vi "openCOMports.vi"(1 "COM Port":refnum<visa-resource-name>="COM8", 2 "index":i32) -> (0 "opened COM port":refnum<visa-resource-name>="COM8")   [LabVIEW 2015]
uses:
  <vilib>/Instr/_visa.llb/VISA Configure Serial Port (Instr).vi
panel:
  in  "Comms":T1(array[cluster])=[{"baud rate "=500000, "data bits "=8, "parity "=enum."None", "flow control "=0, "timeout "=10000, "stop bits "=10}, {"baud rate "=57600, "data bits "=8, "parity "=enum."None", "flow control "=0, "timeout "=10000, "stop bits "=10}] {"stop bits" items=["1.0"=10, "1.5"=15, "2.0"=20]; "flow control" items=["None", "XON/XOFF", "RTS/CTS", "XON/XOFF & RTS/CTS", "DTR/DSR", "XON/XOFF & DTR/DSR"]}
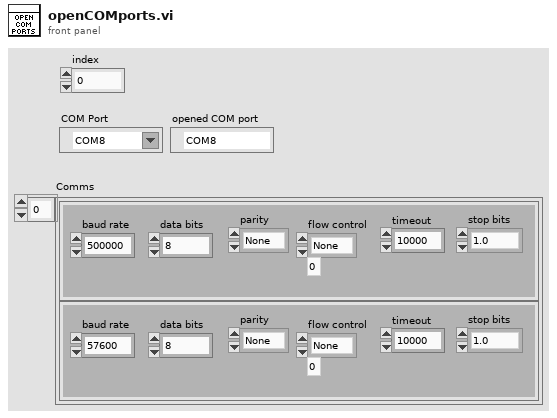
[diagram p1: front panel]
types:
  T1 = cluster{"baud rate ":u32, "data bits ":u16, "parity ":enum16{"None", "Odd", "Even", "Mark", "Space"}, "flow control ":u16, "timeout ":u32, "stop bits ":u16}[]
  T2 = cluster{"baud rate ":u32, "data bits ":u16, "parity ":enum16{"None", "Odd", "Even", "Mark", "Space"}, "flow control ":u16, "timeout ":u32, "stop bits ":u16}
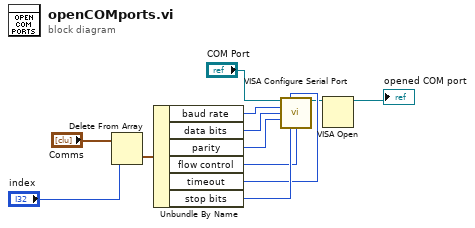
[diagram p0: block diagram]
diagram:
  n1 = Delete From Array(array="Comms", index="index") -> (deleted portion=w5:T2)  [unwired: 1 in, 1 out]
  n2 = Unbundle By Name(w5) -> ("baud rate"=w7:u32, "data bits"=w8:u16, "parity"=w9:enum16{"None", "Odd", "Even", "Mark", "Space"}, "flow control"=w10:u16, "timeout"=w11:u32, "stop bits"=w12:u16)
  n3 = call-poly "VISA Configure Serial Port"("VISA resource name"="COM Port", "timeout (10sec)"=w11, "baud rate (9600)"=w7, "data bits (8)"=w8, "parity (0:none)"=w9, "stop bits (10: 1 bit)"=w12, "flow control (0:none)"=w10) -> ("VISA resource name out"=w6:refnum<visa-resource-name>)  [unwired: 7 in, 1 out]
  n4 = VISA Open(VISA resource name=w6) -> (VISA resource name=→"opened COM port":refnum<visa-resource-name>)  [unwired: 4 in, 1 out]
